vi "init odor descrip array (sub-vi).vi"(8 "error in (no error)":errorcluster, 10 "num odors (10)":i32=10, 11 "array refnum":refnum<vi>) -> (0 "error out":errorcluster, 3 "array refnum out":refnum<vi>)   [LabVIEW 2021]
uses:
  type-defs/odor info cluster (type def).ctl
  type-defs/odor selection (type def).ctl
  type-defs/odor color (type def).ctl
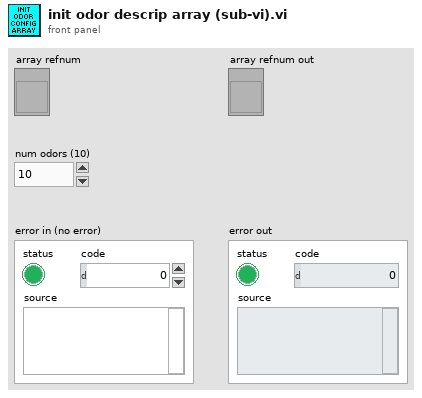
[diagram p1: front panel]
types:
  T1 = typedef "odor info cluster (type def).ctl" = cluster{"odor channel":T2, "odor description":string, "odor color":T3, "odor channel active":bool}
  T2 = typedef "odor selection (type def).ctl" = enum16{"[none]", "odor 1", "odor 2", "odor 3", "odor 4", "odor 5", "odor 6", "odor 7", "odor 8", "odor 9", "odor 10"}
  T3 = typedef "odor color (type def).ctl" = u16
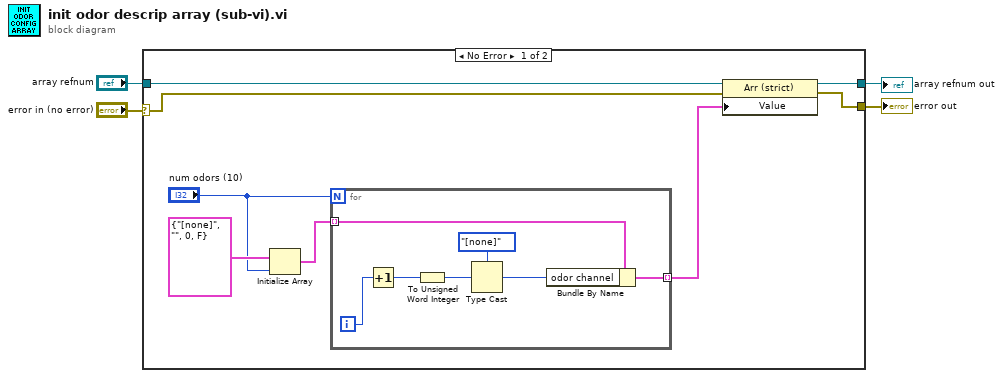
[diagram p0: block diagram]
diagram:
  n1 = case shown="No Error" "error in (no error)" {
    selector: "error in (no error)" -> [w6 w20]
    tunnel: "array refnum" -> [w9 w21]
    tunnel: [w8 w21] -> w3
    tunnel: [w7 w20] -> w2
    frame No Error {
      n2 = Initialize Array(T1 {"odor channel"=enum."[none]", "odor description"="", "odor color"=0, "odor channel active"=FALSE} ("odor description cluster"), "num odors (10)") -> (w11:T1[])
      n3 = for {
        N: "num odors (10)" -> [_]
        tunnel: w11 -> [w19] mode=indexing
        tunnel: [w14] -> w5 mode=indexing
        i -> [w18]
        n4 = Increment(x=w18) -> (x+1=w16:i32)
        n5 = To Unsigned Word Integer(number=w16) -> (unsigned 16bit integer=w13:u16)
        n6 = Type Cast(type=odor_selection_(type_def)."[none]" ("odor channel"), x=w13) -> (*(type *) &x=w15:T2)
        n7 = Bundle By Name(cluster=w19, "odor channel"=w15) -> (w14:T1)
      }
      n8 = property class="Arr (strict)"(reference=w9, error in=w6, "Value"=w5) -> (reference out=w8:refnum<vi>, error out=w7:errorcluster)
    }
    frame Error {
    }
  }
  "array refnum out" <- w3
  "error out" <- w2
